vi "Main Release.vi"(8 "error in":errorcluster, 11 "Main Data Buffer":T1) -> (0 "error out":errorcluster)   [LabVIEW 2020, in "SECS Bridge.lvlib"]
uses:
  SECS Bridge.lvlib
  Main Data Buffer.ctl
  SECS Communication/HSMS Class/HSMS Class.lvclass
  SECS Communication/SECS Data Class/SECS Data Class.lvclass
  SECS Scenarios/Scenarios Class/Scenarios Class.lvclass
  PPL/Universal Function.lvlibp
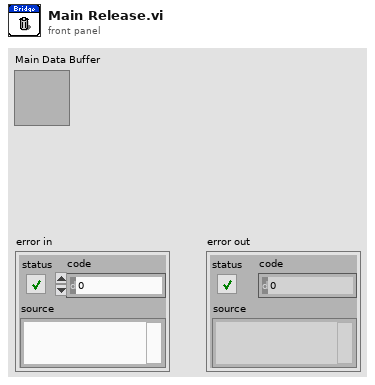
[diagram p1: front panel]
types:
  T1 = typedef "SECS Bridge.lvlib/Main Data Buffer.ctl" = cluster{"HSMS Class":refnum<class "HSMS Class.lvclass">, "SECS Data Class":refnum<class "SECS Data Class.lvclass">, "Scenarios Class":refnum<class "Scenarios Class.lvclass">, "VI Refnum":refnum<vi>, "Ctl Refnum Map":map{string, refnum<vi>}, "Timeout":i32, "Notifier Data":string[], "Event Refnum":refnum<event-registration>}
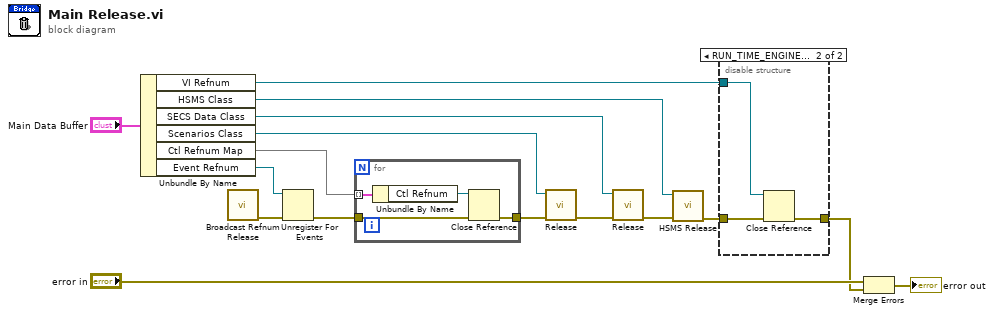
[diagram p0: block diagram]
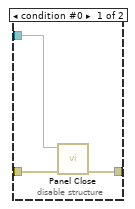
[diagram p2: hidden frame]
diagram:
  n1 = Unbundle By Name("Main Data Buffer") -> ("VI Refnum"=w11:refnum<vi>, "HSMS Class"=w14:refnum<class "HSMS Class.lvclass">, "SECS Data Class"=w15:refnum<class "SECS Data Class.lvclass">, "Scenarios Class"=w3:refnum<class "Scenarios Class.lvclass">, "Ctl Refnum Map"=w5:map{string, refnum<vi>}, "Event Refnum"=w6:refnum<event-registration>)
  n2 = call "Broadcast Refnum Release.vi"() -> ("error out"=w1:errorcluster)  [unwired: 11 in]
  n3 = Unregister For Events(event registration refnum=w6, error in=w1) -> (error out=w7:errorcluster)
  n4 = for {
    tunnel: w5 -> [w20] mode=indexing
    tunnel: [w19] -> w4
    tunnel: w7 -> [w17]
    n5 = Unbundle By Name(w20) -> ("Ctl Refnum"=w18:refnum<vi>)
    n6 = Close Reference(reference=w18, error in (no error)=w17) -> (error out=w19:errorcluster)
  }
  n7 = call "Release.vi"("error in (no error)"=w4, "Scenarios Class in"=w3) -> ("error out"=w2:errorcluster)  [unwired: 9 in]
  n8 = call "Release.vi"("error in (no error)"=w2, "SECS Data Class in"=w15) -> ("error out"=w13:errorcluster)  [unwired: 9 in]
  n9 = call "HSMS Release.vi"("error in (no error)"=w13, "HSMS Class in"=w14) -> ("error out"=w12:errorcluster)  [unwired: 9 in]
  n10 = disable-structure shown="RUN_TIME_ENGINE==False" {
    disable-tunnel: w12 -> [w23 w26]
    disable-tunnel: w11 -> [w22 w24]
    disable-tunnel: [w21 w25] -> w9
    frame condition #0 {
      n11 = call "Panel Close.vi"("error in"=w23, "VI Refnum"=w22) -> ("error out"=w21:errorcluster)  [unwired: 9 in]
    }
    frame condition #1 (active) {
      n12 = Close Reference(reference=w24, error in (no error)=w26) -> (error out=w25:errorcluster)
    }
  }
  n13 = Merge Errors("error in", w9) -> (→"error out":errorcluster)
